vi "ResultsDB Insert Results Data.vi"(6 "Results NameList":string, 7 "Total_OK/NG":string, 8 "error in (no error)":errorcluster, 9 "Results List":string, 10 "StationName":string, 11 "MainBarcode":string) -> (0 "error out":errorcluster, 3 "CMD":string)   [LabVIEW 2021, in "SQLite.lvclass"]
doc: "写入每一步的测试结果到Results表格。\n写入原理：先检测已经保存了几个结果数据，然后依次附加到结果数据列上。\n# 2020-6-8 14:05:45"
uses:
  SQLite.lvclass
  Y:/UTP_2023/Source_Public/DataBase/Top DB/Top DB.lvclass
  <vilib>/Utility/error.llb/Trim Whitespace.vi
  SQLite.lvclass/SQLite.ctl
  <userlib>/LabSQL/LabSQL.lvlib
  vi.lib_New/TopPath/TopPath.lvlib
  <userlib>/sushu/sushu.lvlib
panel:
  out "Update CMD 3":string
  out "Update CMD 2":string
  out "Update CMD":string
  out "EmptyResultColumnIndex":i32
  out "FirstRow":string[](array[string])
  out "source":string
  out "match substring":string
  out "number (0 to 1)":dbl
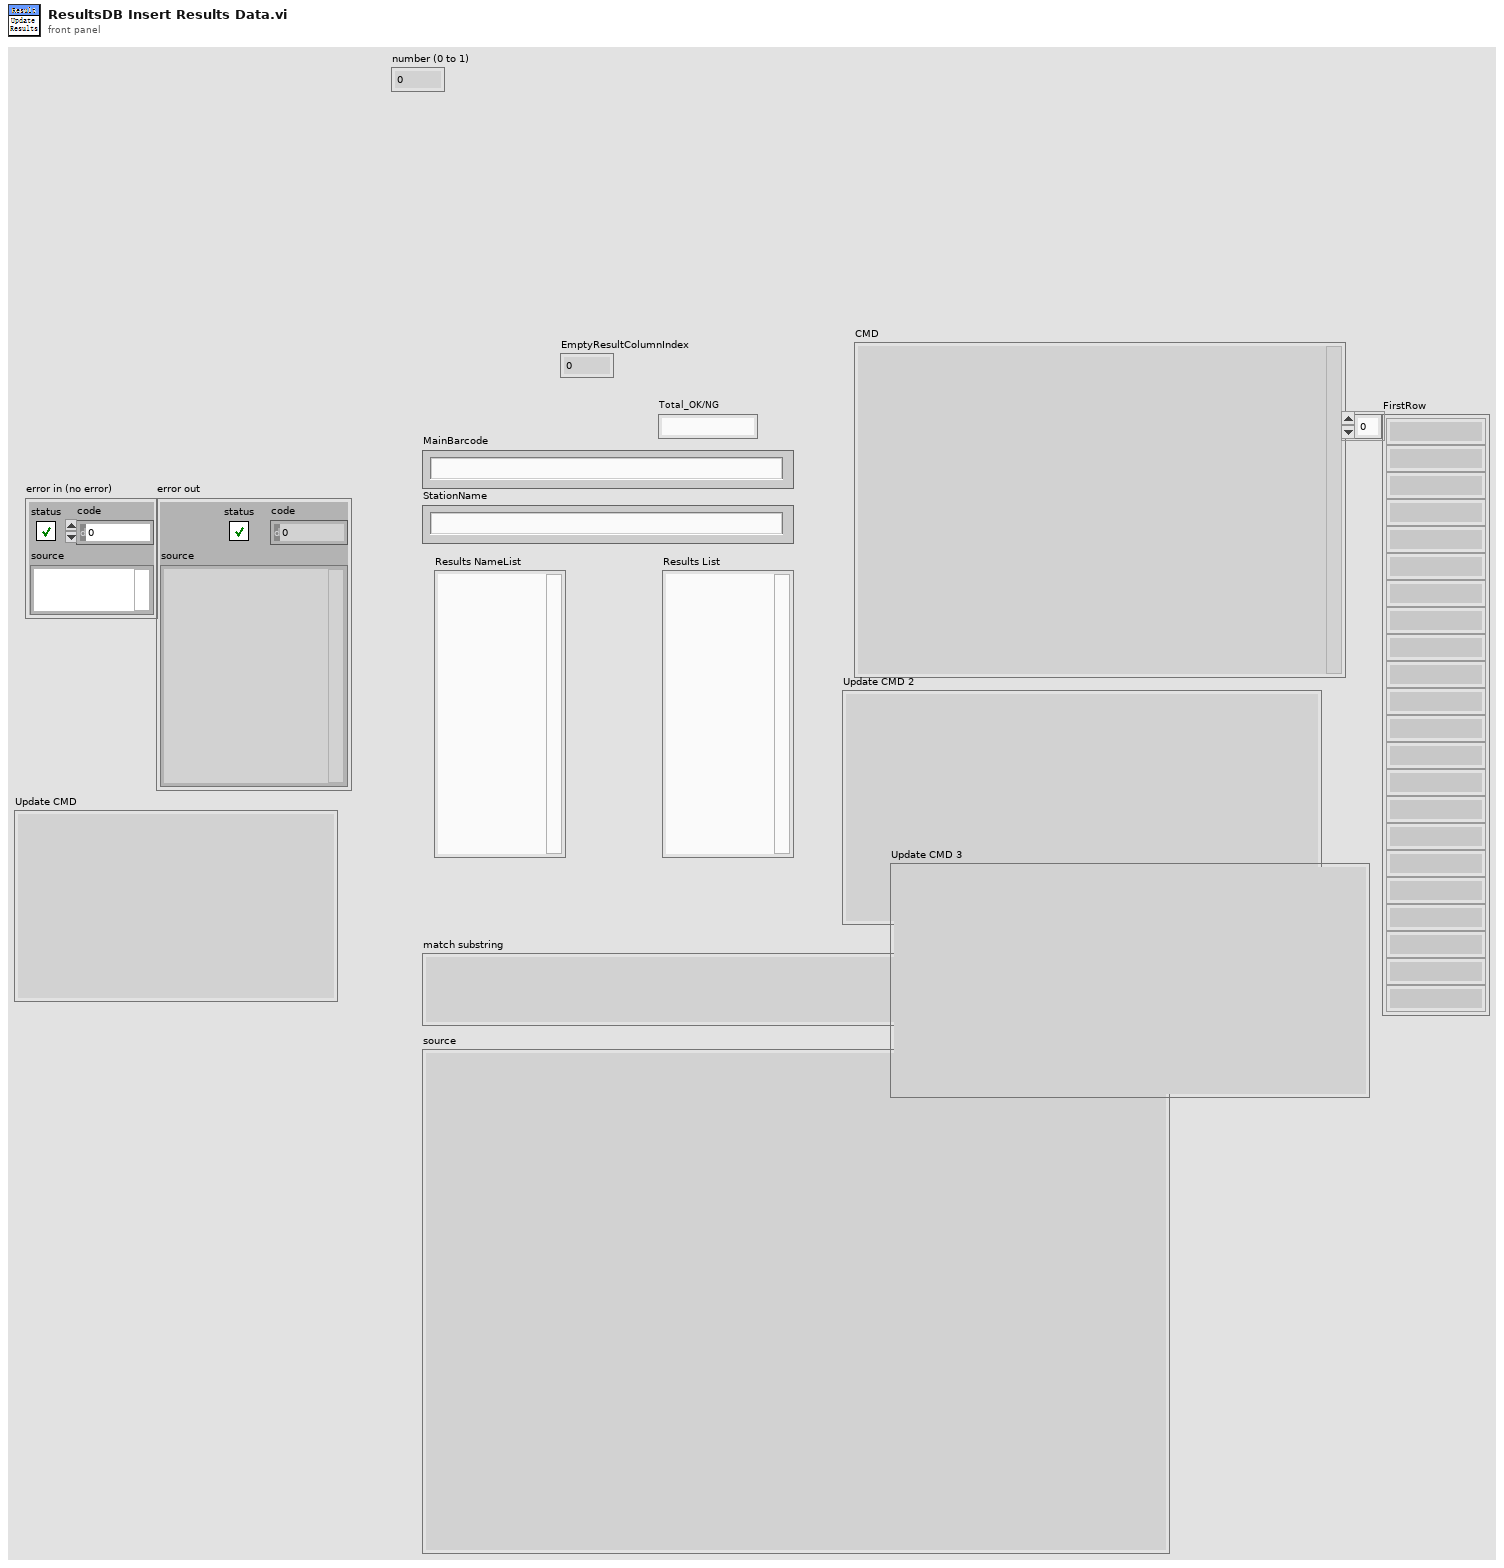
[diagram p1: front panel]
types:
  T1 = cluster{"Core":cluster{"Current VI Reference":refnum<vi>, "Close Panel on Exit?":bool}, "VI Name":string, "Row Numbers":string, "Update?":bool, "CMD":string, "ResultStartindex":i32, "EmptyResultColumnIndex":i32}
  T2 = enum16{"Other", "SQL2008", "SQLite", "Access", "MySQL"}
  T3 = typedef "TopPath.lvlib/Top Path.ctl" = cluster{"LV Source":path, "FilePath":path, "Data":path}
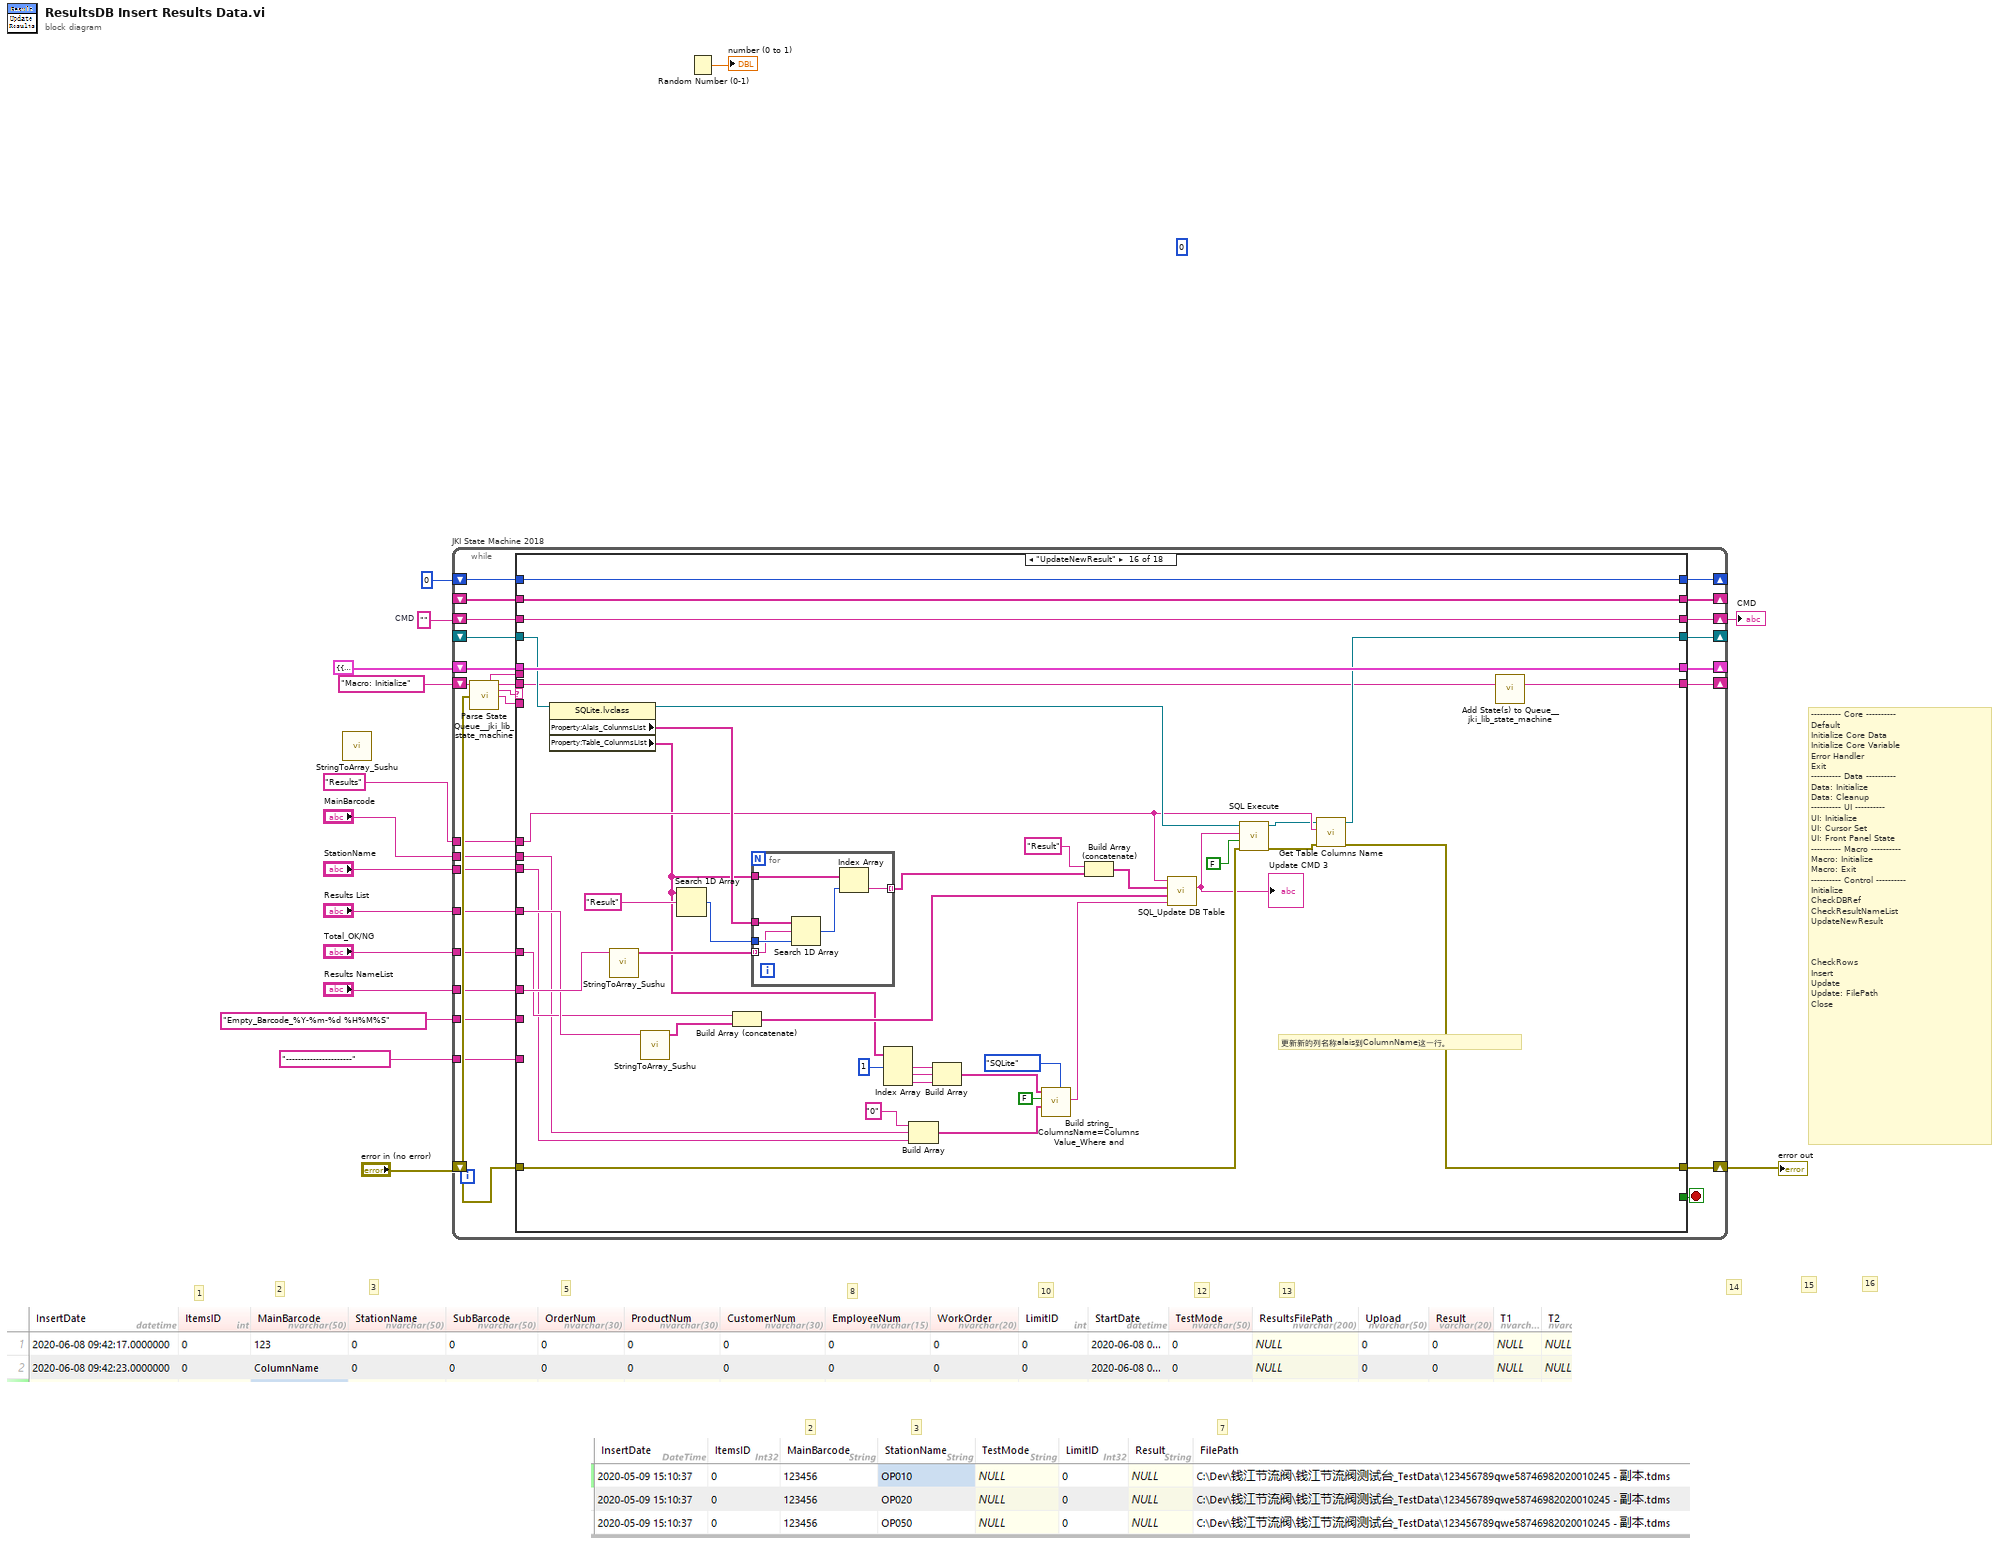
[diagram p0: block diagram]
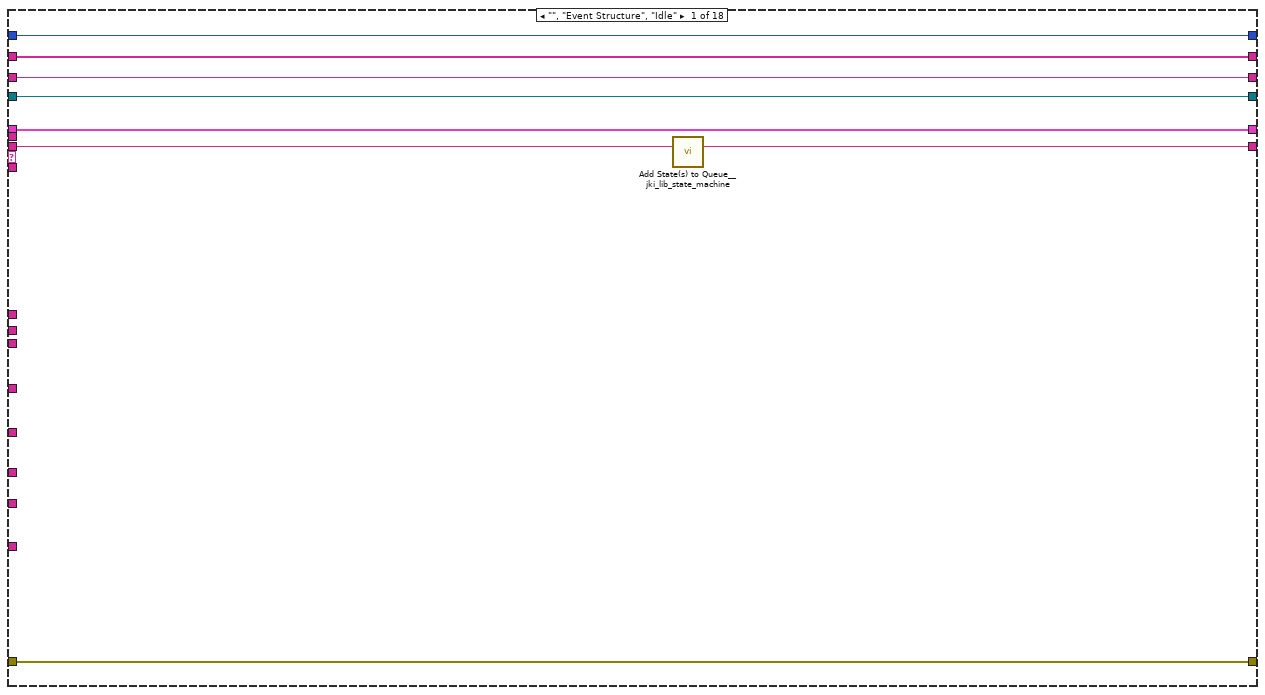
[diagram p2: hidden frame]
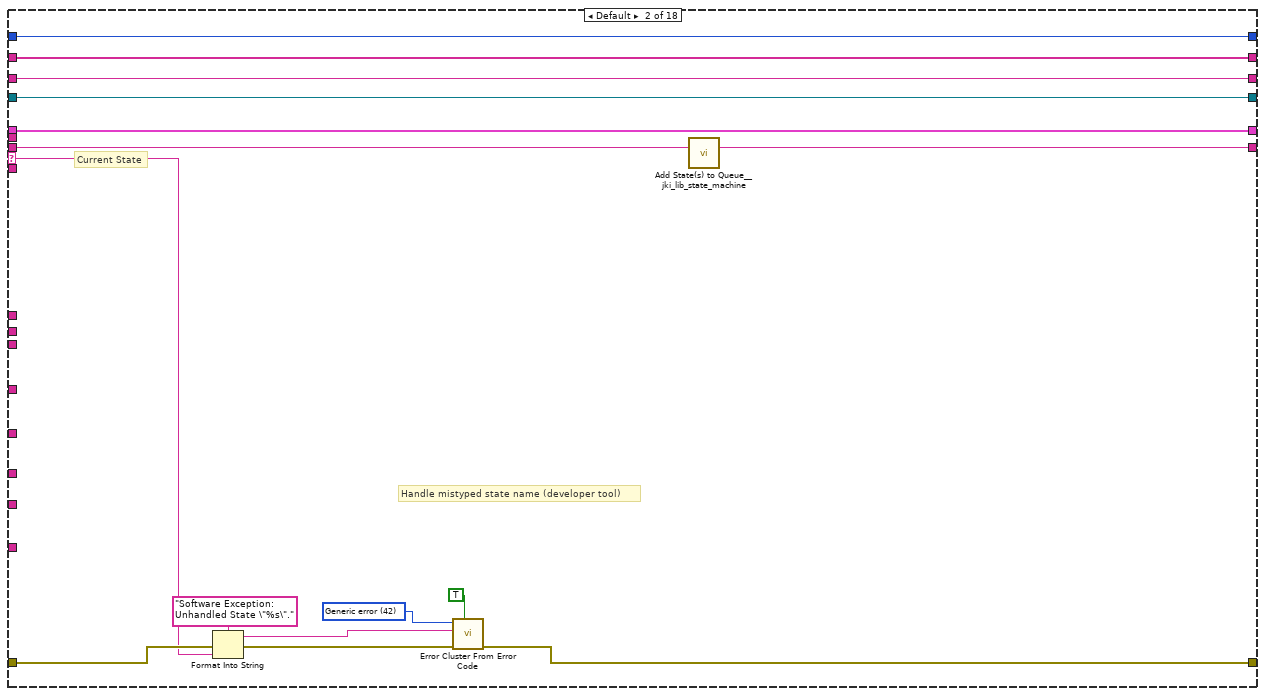
[diagram p3: hidden frame]
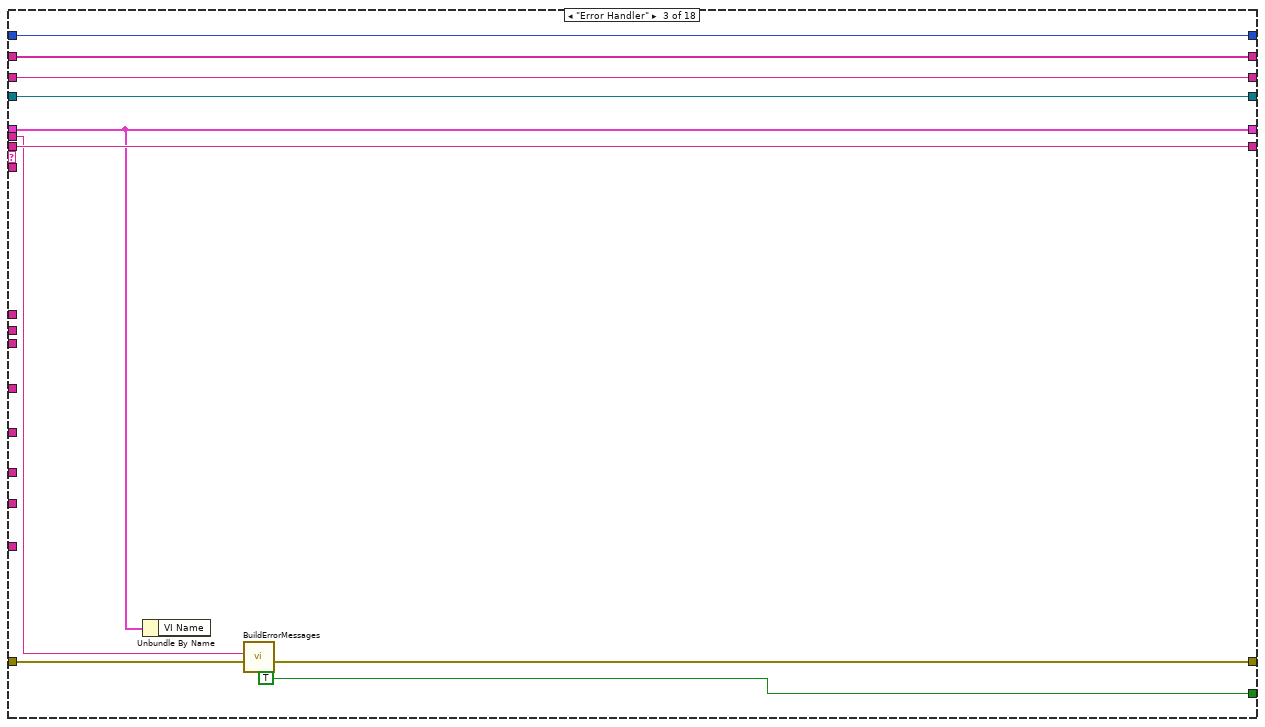
[diagram p4: hidden frame]
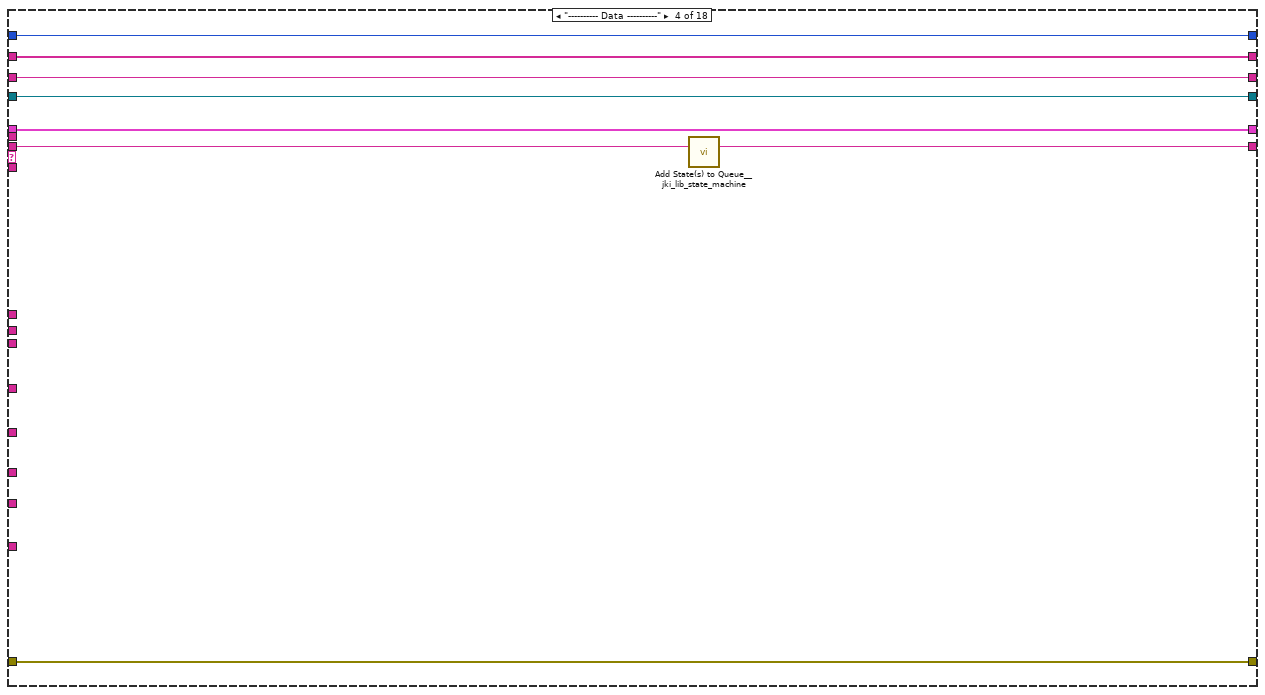
[diagram p5: hidden frame]
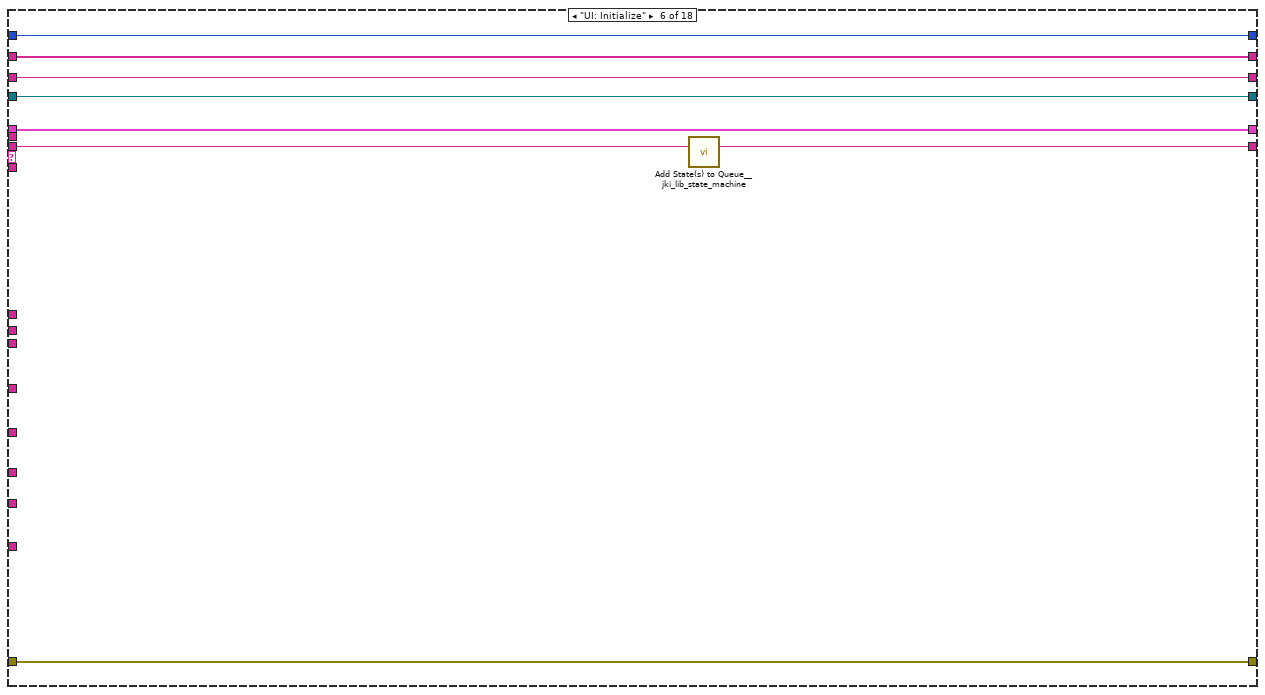
[diagram p7: hidden frame]
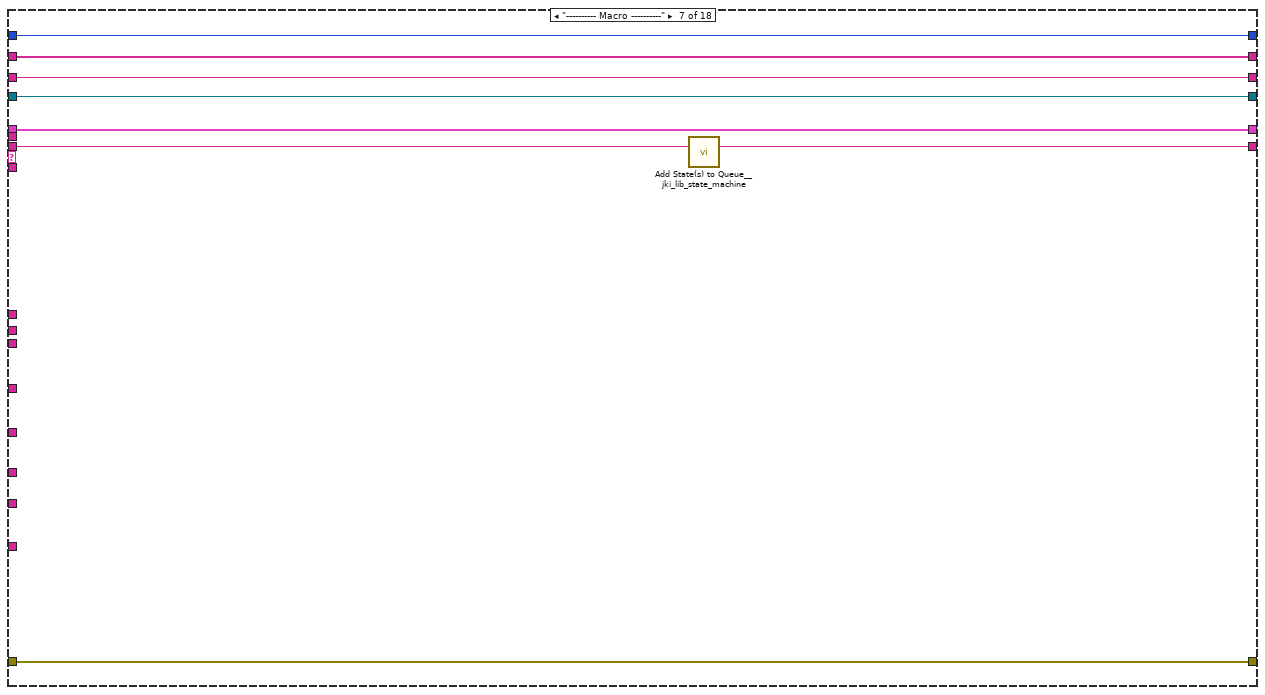
[diagram p8: hidden frame]
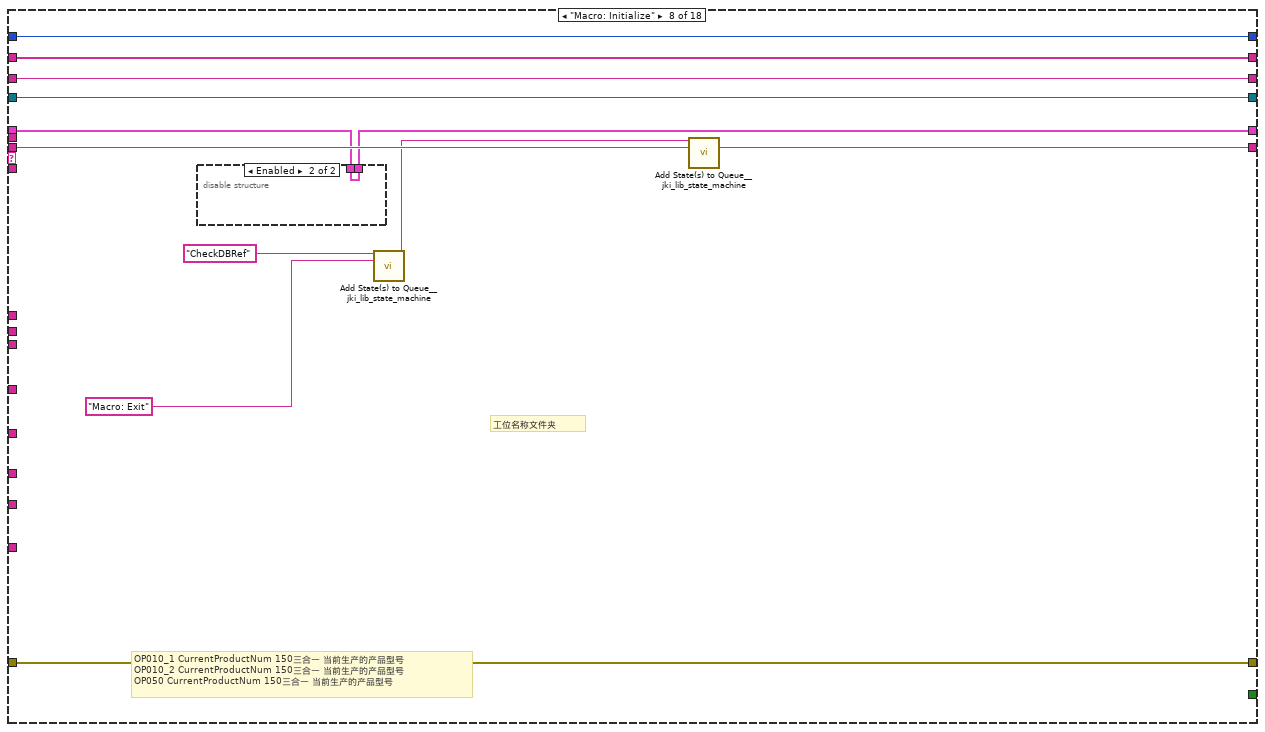
[diagram p9: hidden frame]
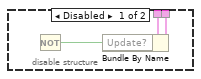
[diagram p10: hidden frame]
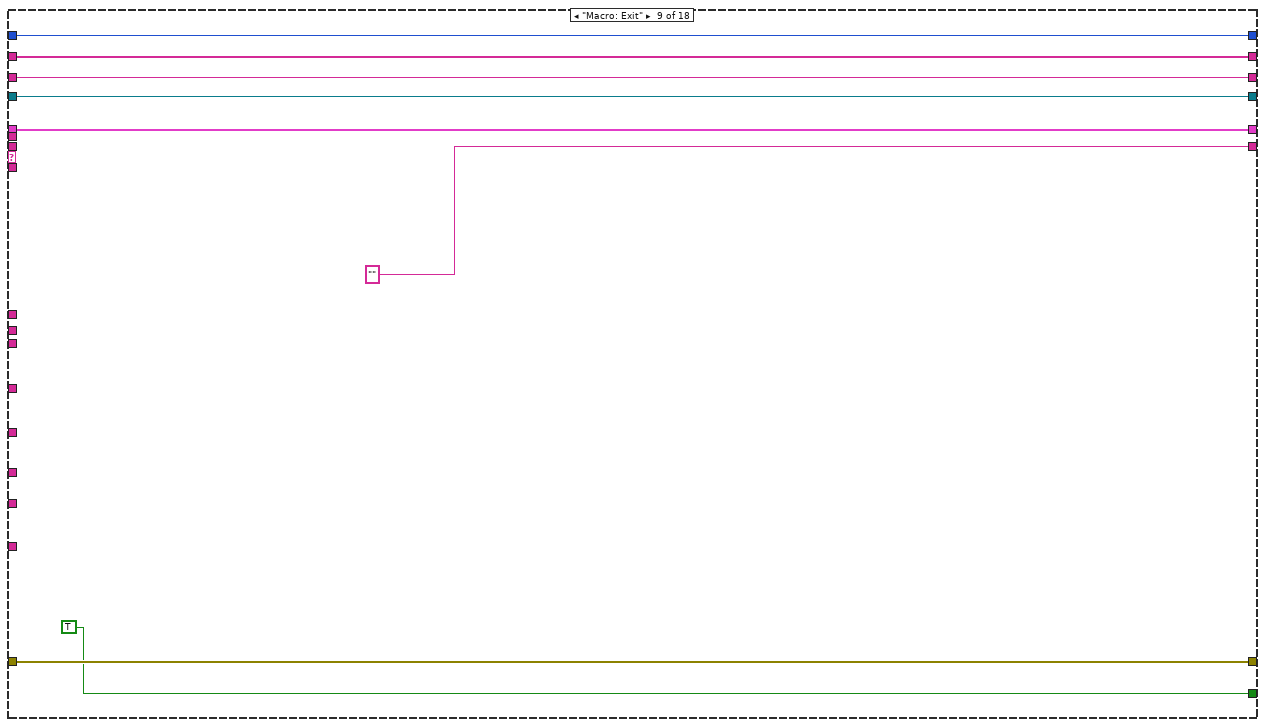
[diagram p11: hidden frame]
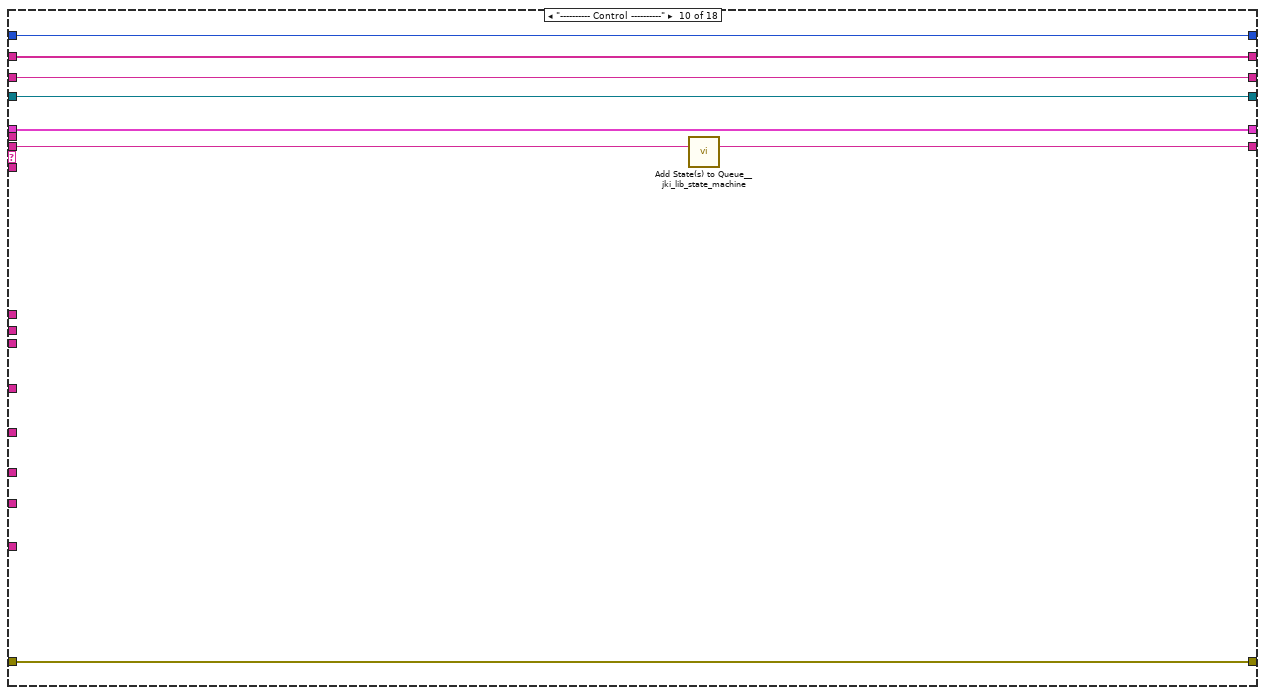
[diagram p12: hidden frame]
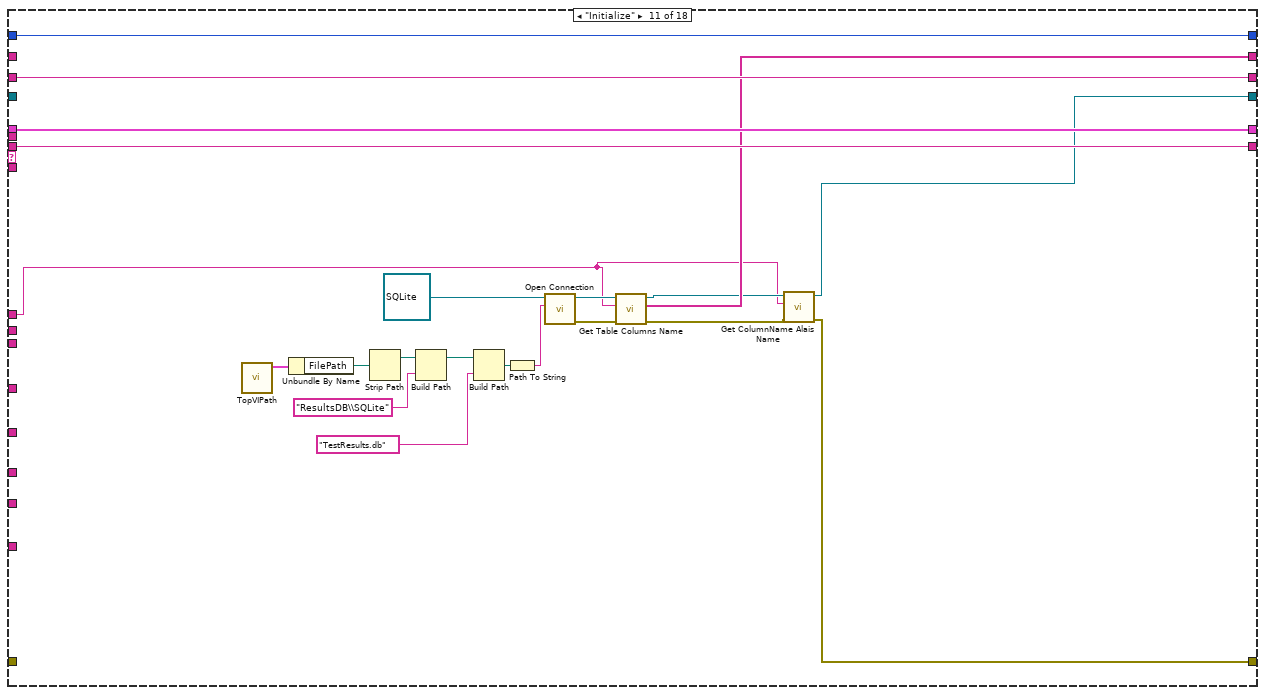
[diagram p13: hidden frame]
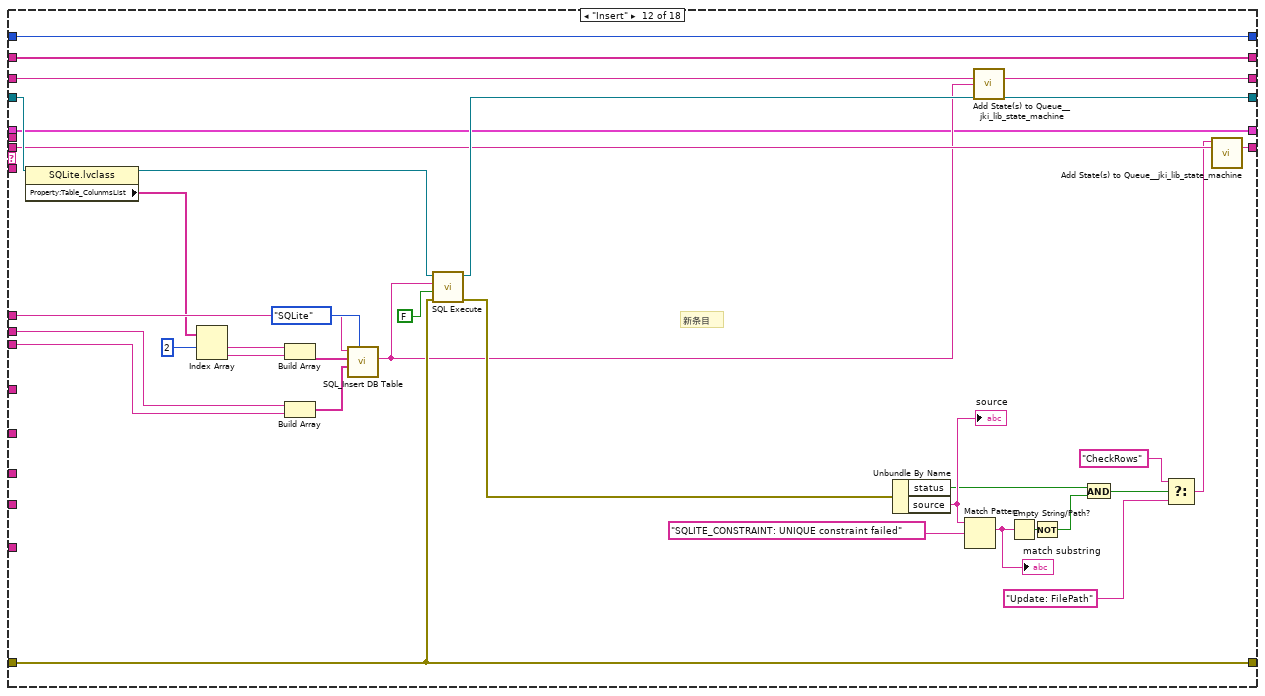
[diagram p14: hidden frame]
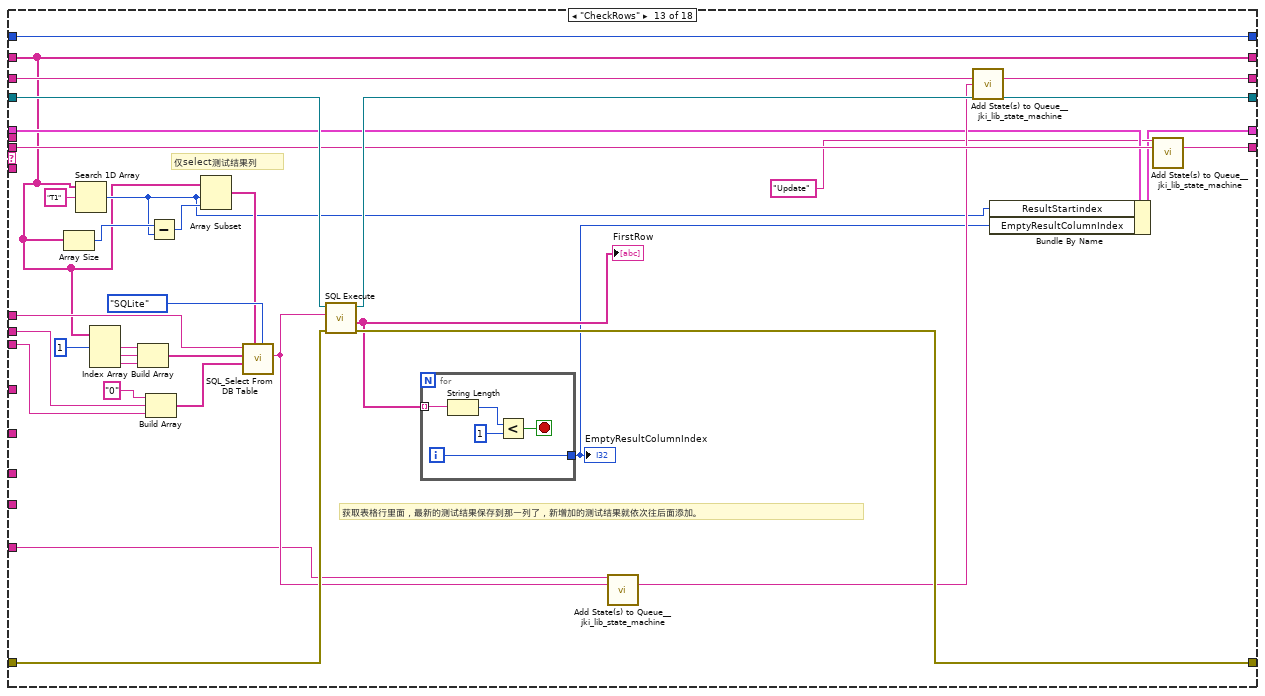
[diagram p15: hidden frame]
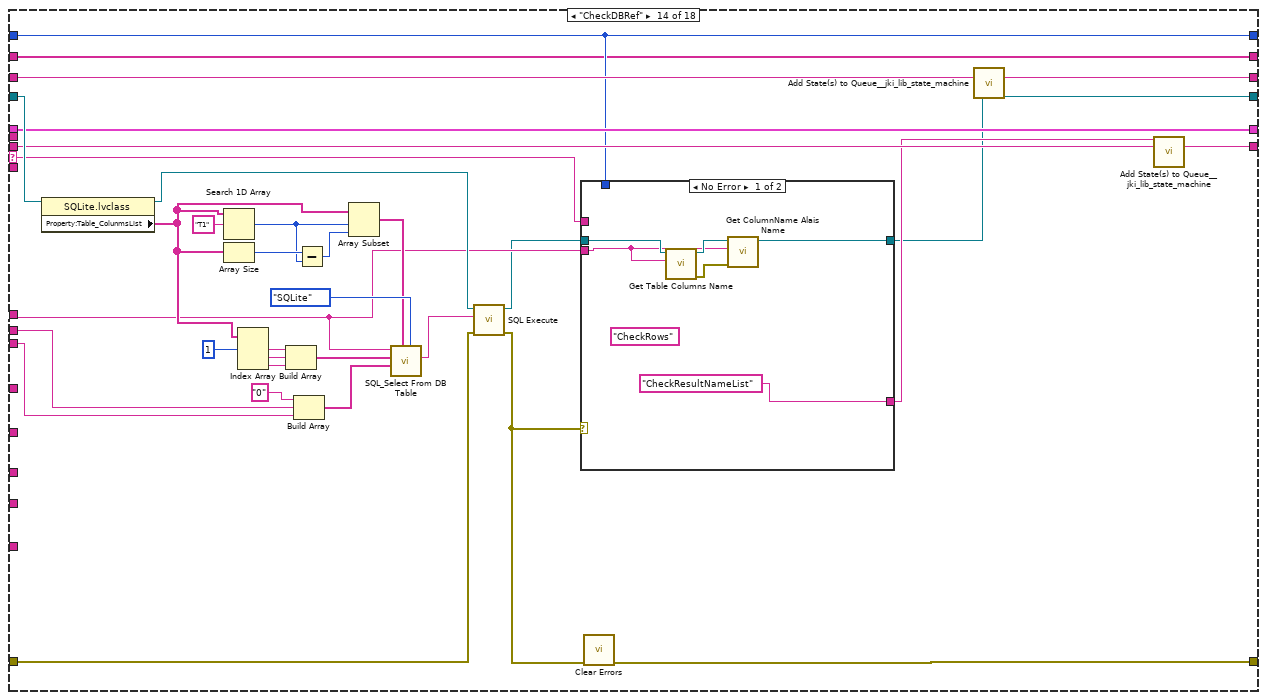
[diagram p16: hidden frame]
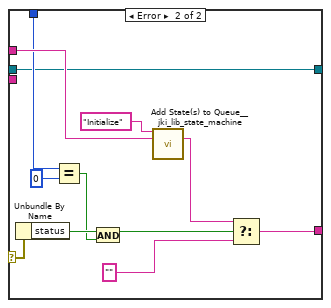
[diagram p17: hidden frame]
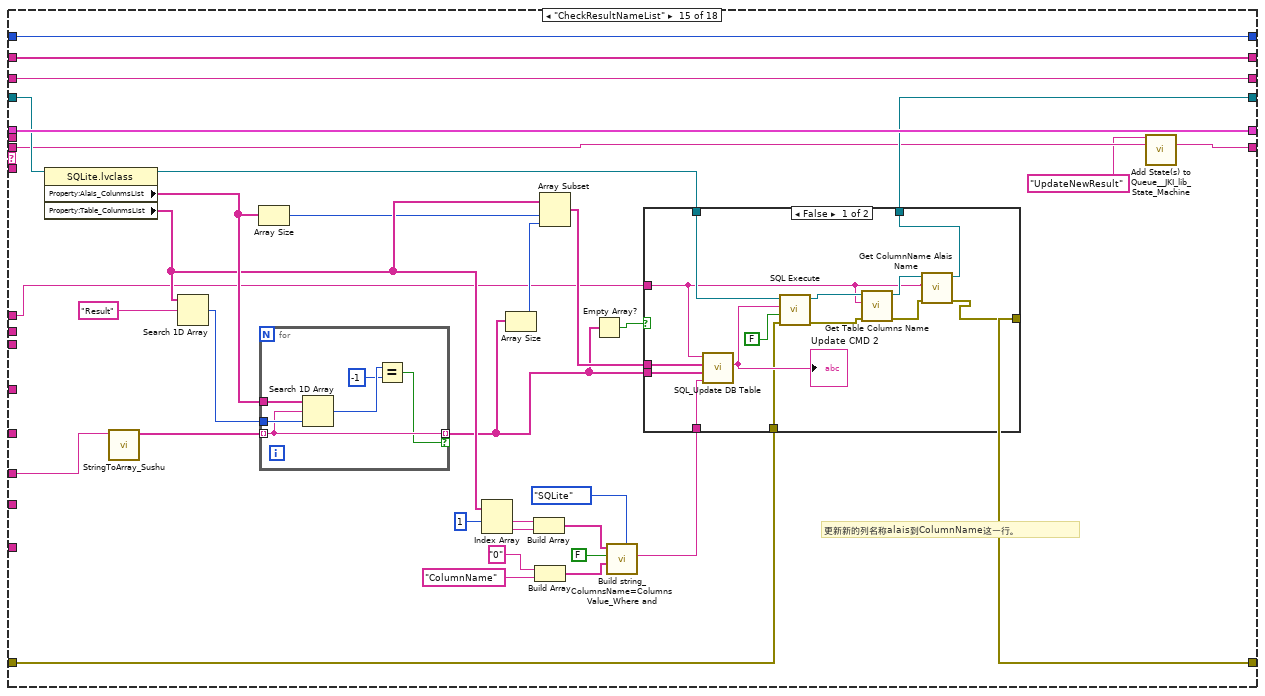
[diagram p18: hidden frame]
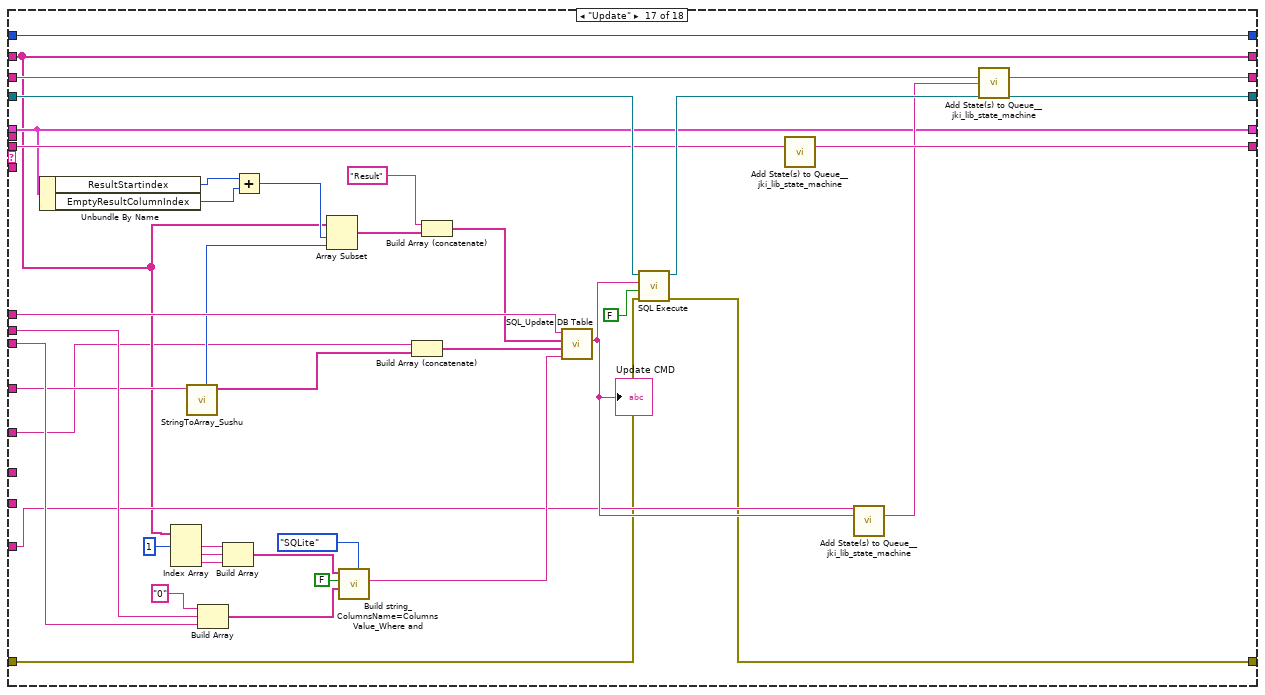
[diagram p20: hidden frame]
diagram:
  w9 = ""  # CMD
  (unwired) 0 ("index (row)")
  # "16"
  # "15"
  # "14"
  # "13"
  # "12"
  # "10"
  # "8"
  # "5"
  # "3"
  # "2"
  # "1"
  # "---------- Core ----------\nDefault\nInitialize Core Data\nInitialize Core Variable\nError Handler\nExit\n---------- Data ----------\nData: Initialize\nData: Cleanup\n---------- UI ----------\nUI: Initialize\nUI: Cursor Set\nUI: Front Panel State\n---------- Macro ----------\nMacro: Initialize\nMacro: Exit\n---------- Control ----------\nInitialize\nCheckDBRef\nCheckResultNameList\nUpdateNewResult\n\n\n\nCheckRows\nInsert\nUpdate\nUpdate: FilePath\nClose"
  # "7"
  # "3"
  # "2"
  n1 = call <userlib>:"StringToArray_Sushu.vi"() -> ()  [unwired: 8 in, 4 out]
  n2 = while "JKI State Machine 2018" {
    shift-right: [w37] -> _
    shift-left: T1 {"Core"={"Current VI Reference"=refnum, "Close Panel on Exit?"=FALSE}, "VI Name"="", "Row Numbers"="", "Update?"=FALSE, "CMD"="", "ResultStartindex"=0, "EmptyResultColumnIndex"=0} ("Data") -> [w36]
    shift-right: [w40] -> w3
    shift-left: "error in (no error)" -> [w35]
    shift-right: [w39] -> _
    shift-left: "Macro: Initialize" -> [w41]
    shift-right: [w33] -> _
    shift-left: _ -> [w34]
    tunnel: "StationName" -> [w31]
    tunnel: "MainBarcode" -> [w30]
    tunnel: "Results" ("TableName") -> [w29]
    tunnel: "Empty_Barcode_%Y-%m-%d %H%M%S" ("time format string (%c)") -> [w28]
    shift-right: [w27] -> w7
    shift-left: w9 -> [w26]
    tunnel: "----------------------" ("State(s) in (\"\")") -> [w25]
    tunnel: "Results List" -> [w24]
    shift-right: [w22] -> _
    shift-left: _ -> [w23]
    shift-right: [w21] -> _
    shift-left: 0 ("y") -> [w20]
    tunnel: "Total_OK/NG" -> [w19]
    tunnel: "Results NameList" -> [w17]
    stop <- w38 stop-if-true
    n3 = call <vilib>:"Parse State Queue__jki_lib_state_machine.vi"("State Queue"=w41, "Error In (no error)"=w35) -> ("Previous State"=w18:string, "Remaining States"=w43:string, "Current State"=w32:string, "Arguments"=w42:string)  [unwired: 10 in]
    n4 = case shown="\"UpdateNewResult\"" w32 {
      selector: w32 -> [_ w56 _ _ _ _ _ _ _ _ _ _ _ w244 _ _ _ _]
      tunnel: w43 -> [w51 w60 w75 w84 w88 w99 w107 w119 _ w139 w160 w172 w216 w257 w287 w366 w420 w436]
      tunnel: w42 -> [_ _ _ _ _ _ _ _ _ _ _ _ _ _ _ _ _ _]
      tunnel: w36 -> [w48 w58 w73 w81 w89 w97 w104 w115 w130 w136 w159 w165 w202 w246 w319 w382 w403 w435]
      tunnel: [w49 w62 w70 w82 w91 w96 w105 w116 w131 w137 w140 w182 w214 w240 w292 w369 w395 w430] -> w40
      tunnel: w35 -> [w49 w61 w71 w82 w91 w96 w105 w116 w131 w137 _ w182 w215 w256 w310 w373 w396 w431]
      tunnel: [w50 w59 w75 w83 w88 w98 w106 w118 "" w138 w160 w173 w217 w258 w288 w367 w421 w436] -> w39
      tunnel: [_ _ TRUE _ _ _ _ _ TRUE _ _ _ _ _ _ _ _ _] -> w38
      tunnel: [w48 w58 w73 w81 w89 w97 w104 w111 w130 w136 w159 w165 w199 w246 w319 w382 w403 w435] -> w37
      tunnel: w34 -> [w47 w55 w74 w80 w90 w95 w103 w117 w129 w135 _ w185 w219 w259 w318 w381 w424 w429]
      tunnel: [w47 w55 w74 w80 w90 w95 w103 w117 w129 w135 w143 w184 w218 w234 w293 w370 w423 w428] -> w33
      tunnel: w18 -> [_ _ w72 _ _ _ _ _ _ _ _ _ _ _ _ _ _ _]
      tunnel: w31 -> [_ _ _ _ _ _ _ _ _ _ _ w186 w220 w260 _ w342 w425 _]
      tunnel: w30 -> [_ _ _ _ _ _ _ _ _ _ _ w187 w221 w261 _ w343 w426 _]
      tunnel: w29 -> [_ _ _ _ _ _ _ _ _ _ w142 w188 w222 w236 w291 w368 w427 _]
      tunnel: w28 -> [_ _ _ _ _ _ _ _ _ _ _ _ _ _ _ _ _ _]
      tunnel: w26 -> [w46 w54 w69 w79 w87 w94 w102 w112 w126 w134 w158 w168 w212 w254 w317 w380 w408 w434]
      tunnel: [w46 w54 w69 w79 w87 w94 w102 w112 w126 w134 w158 w167 w213 w255 w317 w380 w409 w434] -> w27
      tunnel: w25 -> [_ _ _ _ _ _ _ _ _ _ _ _ w209 _ _ _ w405 _]
      tunnel: w24 -> [_ _ _ _ _ _ _ _ _ _ _ _ _ _ _ w361 w404 _]
      tunnel: w23 -> [w45 w53 w68 w78 w86 w93 w101 w109 w125 w133 _ w162 w196 w238 w316 w379 w394 w433]
      tunnel: [w45 w53 w68 w78 w86 w93 w101 w109 w125 w133 w145 w162 w196 w238 w316 w379 w394 w433] -> w22
      tunnel: w20 -> [w44 w52 w67 w77 w85 w92 w100 w108 w124 w132 w146 w164 w195 w243 w315 w378 w393 w432]
      tunnel: [w44 w52 w67 w77 w85 w92 w100 w108 w124 w132 w146 w164 w195 w243 w315 w378 w393 w432] -> w21
      tunnel: w19 -> [_ _ _ _ _ _ _ _ _ _ _ _ _ _ _ w359 w391 _]
      tunnel: w17 -> [_ _ _ _ _ _ _ _ _ _ _ _ _ _ w294 w371 _ _]
      frame "", "Event Structure", "Idle" {
        n5 = call <vilib>:"Add State(s) to Queue__jki_lib_state_machine.vi"("State(s) in (\"\")"=w51) -> ("States Out"=w50:string)  [unwired: 14 in]
      }
      frame Default {
        w65 = 42 items=["No error", "Argument error", "Memory is full", "Out of zone", "End of file", "File already open", "Generic file I/O error", "File not found", "File permission error", "Disk is full", "Duplicate path", "Too many files open", "System feature not enabled", "Resource file not found", "Cannot add resource", "Resource not found", "Image not found", "Image memory error", "Pen does not exist", "Config type invalid", "Config token not found", "Config parse error", "Config memory error", "Bad external code format", "Bad external code offset", "External code not present", "Null window", "Destroy window error", "Null menu", "Print aborted", "Bad print record", "Print driver error", "Windows error during printing", "Memory error during printing", "Print dialog error", "Generic print error", "Invalid device refnum", "Device not found", "Device parameter error", "Device unit error", "Cannot open device", "Device call aborted", "Generic error", "Cancelled by user", "Object ID too low", "Object ID too high", "Object not in heap", "Unknown heap", "Unknown object (invalid DefProc)", "Unknown object (DefProc not in table)", "Message out of range", "Invalid (null) method", "Unknown message", "Manager call not supported", "Bad address", "Network operation in progress", "Network operation timed out", "Connection is busy", "Network attribute not supported", "Network error", "Address in use", "System out of memory", "Connection aborted", "Connection refused", "Not connected", "Already connected", "Connection closed", "Initialization error (interapplication manager)", "Bad occurrence", "Wait on unbound occurrence handler", "Occurrence queue overflow", "Datalog type conflict", "Unused", "Unrecognized type (interapplication manager)", "Memory corrupt", "Failed to make temporary DLL", "Old CIN version", "Drag socket not found", "Failed to load drop-object", "Failed to register OLE object", "Failed to release OLE object", "Format specifier type mismatch", "Unknown format specifier", "Too few format specifiers", "Too many format specifiers", "Scan failed", "Newer CIN version", "Error converting to variant", "Runtime menu error", "Password tampered", "Variant attribute not found", "Incompatible variant data type", "Event data is not available", "Event Store is not present", "Occurrence is not found", "Event Queue is not created", "Event info is not available", "Refnum passed is NULL", "Error retrieving Class GUID", "Error retrieving CoClass GUID", "Error retrieving TypeLib GUID.", "Bad built application magic bytes.", "Specific driver is different from the specific driver associated with the Logical Name.", "There is no session opened to the class driver.", "Max Error", "MAX - Error with config objects", "MAX - Error loading configuration", "MAX - Group not supported"]
        # "Current State"
        # "Handle mistyped state name (developer tool)"
        n6 = Format Into String(format string="Software Exception: Unhandled State \"%s\"." ("message"), error in=w61, w56) -> (resulting string=w64:string, error out=w63:errorcluster)  [unwired: 1 in]
        n7 = call <vilib>:"Error Cluster From Error Code.vi"("show call chain? (False)"=TRUE, "error in (no error)"=w63, "error message (\"\")"=w64, "error code (0)"=w65) -> ("error out"=w62:errorcluster)  [unwired: 5 in]
        n8 = call <vilib>:"Add State(s) to Queue__jki_lib_state_machine.vi"("State(s) in (\"\")"=w60) -> ("States Out"=w59:string)  [unwired: 14 in]
      }
      frame "Error Handler" {
        n9 = Unbundle By Name(w73) -> ()  [unwired: 1 out]
        n10 = call <userlib>:"BuildErrorMessages.vi"("error in"=w71, "ErrorCase"=w72) -> ("error out (no error)"=w70:errorcluster)  [unwired: 7 in, 2 out]
      }
      frame "---------- Data ----------" {
        n11 = call <vilib>:"Add State(s) to Queue__jki_lib_state_machine.vi"("State(s) in (\"\")"=w84) -> ("States Out"=w83:string)  [unwired: 14 in]
      }
      frame "Data: Initialize" {
      }
      frame "UI: Initialize" {
        n12 = call <vilib>:"Add State(s) to Queue__jki_lib_state_machine.vi"("State(s) in (\"\")"=w99) -> ("States Out"=w98:string)  [unwired: 14 in]
      }
      frame "---------- Macro ----------" {
        n13 = call <vilib>:"Add State(s) to Queue__jki_lib_state_machine.vi"("State(s) in (\"\")"=w107) -> ("States Out"=w106:string)  [unwired: 14 in]
      }
      frame "Macro: Initialize" {
        # "OP010_1\tCurrentProductNum\t150三合一\t当前生产的产品型号\nOP010_2\tCurrentProductNum\t150三合一\t当前生产的产品型号\nOP050\tCurrentProductNum\t150三合一\t当前生产的产品型号"
        # "工位名称文件夹"
        n14 = disable-structure shown="Enabled" {
          disable-tunnel: w115 -> [w122 w123]
          disable-tunnel: [w121 w123] -> w111
          frame Disabled {
            n15 = Not() -> (.not. x?=w120:bool)  [unwired: 1 in]
            n16 = Bundle By Name(cluster=w122, "Update?"=w120) -> (w121:T1)
          }
          frame Enabled {
          }
        }
        n17 = call <vilib>:"Add State(s) to Queue__jki_lib_state_machine.vi"("State(s) in Front (\"\")"="CheckDBRef" ("State(s) in Front (\"\")"), "State(s) in (\"\")"="Macro: Exit") -> ("States Out"=w114:string)  [unwired: 13 in]
        n18 = call <vilib>:"Add State(s) to Queue__jki_lib_state_machine.vi"("State(s) in Front (\"\")"=w114, "State(s) in (\"\")"=w119) -> ("States Out"=w118:string)  [unwired: 13 in]
      }
      frame "Macro: Exit" {
      }
      frame "---------- Control ----------" {
        n19 = call <vilib>:"Add State(s) to Queue__jki_lib_state_machine.vi"("State(s) in (\"\")"=w139) -> ("States Out"=w138:string)  [unwired: 14 in]
      }
      frame "Initialize" {
        n20 = call "TopVIPath.vi"() -> ("TopPath"=w147:T3)  [unwired: 10 in, 1 out]
        n21 = Unbundle By Name(w147) -> ("FilePath"=w157:path)
        n22 = Strip Path(path=w157) -> (stripped path=w156:path)  [unwired: 1 out]
        n23 = Build Path(base path=w156, name or relative path="ResultsDB\\SQLite") -> (appended path=w154:path)
        n24 = Build Path(base path=w154, name or relative path="TestResults.db") -> (appended path=w152:path)
        n25 = Path To String(path=w152) -> (string=w151:string)
        n26 = call-dynamic "Open Connection.vi"("ConnectionString"=w151, "HostDB in"=refnum<class "SQLite.lvclass"> refnum ("SQLite.lvclass")) -> ("error out"=w149:errorcluster, "HostDB out"=w150:refnum<class "SQLite.lvclass">)  [unwired: 8 in]
        n27 = call-dynamic "Get Table Columns Name.vi"("error in (no error)"=w149, "TableName"=w142, "HostDB in"=w150) -> ("error out"=w141:errorcluster, "Table_ColunmsList"=w145:string[], "HostDB out"=w144:refnum<class "SQLite.lvclass">)  [unwired: 4 in, 2 out]
        n28 = call "Get ColumnName Alais Name.vi"("error in (no error)"=w141, "TableName"=w142, "SQLite in"=w144) -> ("error out"=w140:errorcluster, "SQLite out"=w143:refnum<class "SQLite.lvclass">)  [unwired: 6 in, 1 out]
      }
      frame "Insert" {
        # "新条目"
        n29 = property class="SQLite.lvclass"(reference=w185) -> (reference out=w163:refnum<class "SQLite.lvclass">, "Property:Table_ColunmsList"=w161:string[])  [unwired: 1 in, 1 out]
        n30 = Index Array(array=w161, index #1=2 ("index")) -> (element #1=w193:string, element #2=w194:string)  [unwired: 1 in]
        n31 = Build Array(w193, w194) -> (w191:string[])
        n32 = Build Array(w187, w186) -> (w190:string[])
        n33 = call <userlib>:"SQL_Insert DB Table.vi"("DB Type"=T2."SQLite", "ColumnsValue"=w190, "ColumnsName"=w191, "Table Name"=w188) -> ("Insert DB String"=w166:string)  [unwired: 7 in]
        n34 = call-dynamic "SQL Execute.vi"("error in (no error)"=w182, "Return Data (T)"=FALSE, "Command Text"=w166, "HostDB in"=w163) -> ("error out"=w169:errorcluster, "HostDB out"=w184:refnum<class "SQLite.lvclass">)  [unwired: 3 in, 3 out]
        n35 = Unbundle By Name(w169) -> ("status"=w178:bool, "source"=w181:string)
        "source" <- w181
        n36 = Match Pattern(string=w181, regular expression="SQLITE_CONSTRAINT: UNIQUE constraint failed") -> (match substring=w179:string)  [unwired: 1 in, 3 out]
        "match substring" <- w179
        n37 = call <vilib>:"Add State(s) to Queue__jki_lib_state_machine.vi"("State(s) in (\"\")"=w168, "State(s) at Back (\"\")"=w166) -> ("States Out"=w167:string)  [unwired: 13 in]
        n38 = Empty String/Path?(string/path=w179) -> (empty?=w177:bool)
        n39 = Not(x=w177) -> (.not. x?=w170:bool)
        n40 = And(x=w178, y=w170) -> (x .and. y?=w176:bool)
        n41 = Select(t="CheckRows", s=w176, f="Update: FilePath") -> (s? t:f=w171:string)
        n42 = call <vilib>:"Add State(s) to Queue__jki_lib_state_machine.vi"("State(s) in Front (\"\")"=w171, "State(s) in (\"\")"=w172) -> ("States Out"=w173:string)  [unwired: 13 in]
      }
      frame "CheckRows" {
        # "获取表格行里面，最新的测试结果保存到那一列了，新增加的测试结果就依次往后面添加。"
        # "仅select测试结果列"
        n43 = Array Size(array=w196) -> (size(s)=w205:i32)
        n44 = Search 1D Array(1D array=w196, element="T1") -> (index of element=w198:i32)  [unwired: 1 in]
        n45 = Index Array(array=w196, index #1=1 ("index")) -> (element #1=w227:string, element #2=w228:string, element #3=w208:string)  [unwired: 2 in]
        n46 = Build Array(w227, w228, w208) -> (w225:string[])
        n47 = Build Array("0" ("element"), w221, w220) -> (w224:string[])
        n48 = Subtract(x=w205, y=w198) -> (x-y=w204:i32)
        n49 = Array Subset(array=w196, index=w198, length=w204) -> (w203:string[])
        n50 = call <userlib>:"SQL_Select From DB Table.vi"("DB Type"=T2."SQLite", "SelectedColumnsNameList"=w203, "ColumnsValue"=w224, "ColumnsNameList"=w225, "TableName"=w222) -> ("Select SQL CMD"=w210:string)  [unwired: 6 in]
        n51 = call-dynamic "SQL Execute.vi"("error in (no error)"=w215, "Command Text"=w210, "HostDB in"=w219) -> ("error out"=w214:errorcluster, "FirstRow"=w201:string[], "HostDB out"=w218:refnum<class "SQLite.lvclass">)  [unwired: 4 in, 2 out]
        "FirstRow" <- w201
        n52 = for {
          tunnel: w201 -> [w233] mode=indexing
          tunnel: [w229] -> w197
          i -> [w229]
          stop <- w230 stop-if-true
          n53 = String Length(string=w233) -> (length=w232:i32)
          n54 = Less?(x=w232, y=1) -> (x < y?=w230:bool)
        }
        "EmptyResultColumnIndex" <- w197
        n55 = call <vilib>:"Add State(s) to Queue__jki_lib_state_machine.vi"("State(s) in Front (\"\")"=w209, "State(s) in (\"\")"=w210) -> ("States Out"=w211:string)  [unwired: 13 in]
        n56 = call <vilib>:"Add State(s) to Queue__jki_lib_state_machine.vi"("State(s) in (\"\")"=w212, "State(s) at Back (\"\")"=w211) -> ("States Out"=w213:string)  [unwired: 13 in]
        n57 = Bundle By Name(cluster=w202, "ResultStartindex"=w198, "EmptyResultColumnIndex"=w197) -> (w199:T1)
        n58 = call <vilib>:"Add State(s) to Queue__jki_lib_state_machine.vi"("State(s) in Front (\"\")"="Update" ("State(s) in Front (\"\")"), "State(s) in (\"\")"=w216) -> ("States Out"=w217:string)  [unwired: 13 in]
      }
      frame "CheckDBRef" {
        n59 = property class="SQLite.lvclass"(reference=w259) -> (reference out=w239:refnum<class "SQLite.lvclass">, "Property:Table_ColunmsList"=w237:string[])  [unwired: 1 in, 1 out]
        n60 = Search 1D Array(1D array=w237, element="T1") -> (index of element=w247:i32)  [unwired: 1 in]
        n61 = Array Size(array=w237) -> (size(s)=w249:i32)
        n62 = Index Array(array=w237, index #1=1 ("index")) -> (element #1=w266:string, element #2=w267:string, element #3=w252:string)  [unwired: 2 in]
        n63 = Build Array(w266, w267, w252) -> (w264:string[])
        n64 = Build Array("0" ("element"), w261, w260) -> (w263:string[])
        n65 = Subtract(x=w249, y=w247) -> (x-y=w248:i32)
        n66 = Array Subset(array=w237, index=w247, length=w248) -> (w241:string[])
        n67 = call <userlib>:"SQL_Select From DB Table.vi"("DB Type"=T2."SQLite", "SelectedColumnsNameList"=w241, "ColumnsValue"=w263, "ColumnsNameList"=w264, "TableName"=w236) -> ("Select SQL CMD"=w253:string)  [unwired: 6 in]
        n68 = call-dynamic "SQL Execute.vi"("error in (no error)"=w256, "Command Text"=w253, "HostDB in"=w239) -> ("error out"=w245:errorcluster, "HostDB out"=w235:refnum<class "SQLite.lvclass">)  [unwired: 4 in, 3 out]
        n69 = case shown="No Error" w245 {
          selector: w245 -> [_ w281]
          tunnel: w244 -> [_ w282]
          tunnel: ["CheckResultNameList" ("TableName") w280] -> w242
          tunnel: w243 -> [_ w277]
          tunnel: w235 -> [w271 w274]
          tunnel: w236 -> [w269 _]
          tunnel: [w272 w274] -> w234
          frame No Error {
            (unwired) "CheckRows" ("TableName")
            n70 = call-dynamic "Get Table Columns Name.vi"("TableName"=w269, "HostDB in"=w271) -> ("error out"=w268:errorcluster, "HostDB out"=w270:refnum<class "SQLite.lvclass">)  [unwired: 5 in, 3 out]
            n71 = call "Get ColumnName Alais Name.vi"("error in (no error)"=w268, "TableName"=w269, "SQLite in"=w270) -> ("SQLite out"=w272:refnum<class "SQLite.lvclass">)  [unwired: 6 in, 2 out]
          }
          frame Error {
            n72 = Unbundle By Name(w281) -> ("status"=w279:bool)
            n73 = Equal?(x=w277, y=0) -> (x = y?=w275:bool)
            n74 = And(x=w279, y=w275) -> (x .and. y?=w278:bool)
            n75 = call <vilib>:"Add State(s) to Queue__jki_lib_state_machine.vi"("State(s) in Front (\"\")"="Initialize" ("Remaining States"), "State(s) in (\"\")"=w282) -> ("States Out"=w283:string)  [unwired: 13 in]
            n76 = Select(t=w283, s=w278, f="") -> (s? t:f=w280:string)
          }
        }
        n77 = call <vilib>:"Clear Errors.vi"("error in (no error)"=w245) -> ("error out"=w240:errorcluster)  [unwired: 5 in, 1 out]
        n78 = call <vilib>:"Add State(s) to Queue__jki_lib_state_machine.vi"("State(s) in (\"\")"=w254) -> ("States Out"=w255:string)  [unwired: 14 in]
        n79 = call <vilib>:"Add State(s) to Queue__jki_lib_state_machine.vi"("State(s) in Front (\"\")"=w242, "State(s) in (\"\")"=w257) -> ("States Out"=w258:string)  [unwired: 13 in]
      }
      frame "CheckResultNameList" {
        # "更新新的列名称alais到ColumnName这一行。"
        n80 = property class="SQLite.lvclass"(reference=w318) -> (reference out=w311:refnum<class "SQLite.lvclass">, "Property:Alais_ColunmsList"=w299:string[], "Property:Table_ColunmsList"=w298:string[])  [unwired: 1 in, 1 out]
        n81 = call <userlib>:"StringToArray_Sushu.vi"("State Queue"=w294) -> ("Array"=w314:string[])  [unwired: 7 in, 3 out]
        n82 = Search 1D Array(1D array=w298, element="Result") -> (index of element=w312:i32)  [unwired: 1 in]
        n83 = Array Size(array=w299) -> (size(s)=w297:i32)
        n84 = for {
          tunnel: w314 -> [w337] mode=indexing
          tunnel: w299 -> [w341]
          tunnel: w312 -> [w340]
          tunnel: [w337] -> w290 mode=indexing if=w336
          n85 = Search 1D Array(1D array=w341, element=w337, start index (0)=w340) -> (index of element=w339:i32)
          n86 = Equal?(x=w339, y=-1) -> (x = y?=w336:bool)
        }
        n87 = Index Array(array=w298, index #1=1 ("index")) -> (element #1=w308:string, element #2=w307:string)  [unwired: 1 in]
        n88 = Array Size(array=w290) -> (size(s)=w296:i32)
        n89 = Build Array(w308, w307) -> (w306:string[])
        n90 = Build Array("0" ("element"), "ColumnName" ("element")) -> (w304:string[])
        n91 = Array Subset(array=w298, index=w297, length=w296) -> (w295:string[])
        n92 = Empty Array?(array=w290) -> (empty?=w289:bool)
        n93 = call <userlib>:"Build string_ColumnsName=ColumnsValue_Where and.vi"("DB Type"=T2."SQLite", "ColumnsValue"=w304, "Check ASCII?"=FALSE, "ColumnsNameList"=w306) -> ("ColumnName='ColumnValue'"=w301:string)  [unwired: 7 in]
        n94 = case shown="False" w289 {
          tunnel: w311 -> [w331 w335]
          tunnel: w310 -> [w330 w334]
          tunnel: w301 -> [w329 _]
          tunnel: w295 -> [w328 _]
          tunnel: [w323 w335] -> w293
          tunnel: [w320 w334] -> w292
          tunnel: w291 -> [w322 _]
          tunnel: w290 -> [w325 _]
          frame False {
            n95 = call <userlib>:"SQL_Update DB Table.vi"("where name='value'"=w329, "ColumnsValue"=w325, "ColumnsNameList"=w328, "TableName"=w322) -> ("Update CMD"=w332:string)  [unwired: 7 in]
            "Update CMD 2" <- w332
            n96 = call-dynamic "SQL Execute.vi"("error in (no error)"=w330, "Return Data (T)"=FALSE, "Command Text"=w332, "HostDB in"=w331) -> ("error out"=w326:errorcluster, "HostDB out"=w327:refnum<class "SQLite.lvclass">)  [unwired: 3 in, 3 out]
            n97 = call-dynamic "Get Table Columns Name.vi"("error in (no error)"=w326, "TableName"=w322, "HostDB in"=w327) -> ("error out"=w321:errorcluster, "HostDB out"=w324:refnum<class "SQLite.lvclass">)  [unwired: 4 in, 3 out]
            n98 = call "Get ColumnName Alais Name.vi"("error in (no error)"=w321, "TableName"=w322, "SQLite in"=w324) -> ("error out"=w320:errorcluster, "SQLite out"=w323:refnum<class "SQLite.lvclass">)  [unwired: 6 in, 1 out]
          }
          frame True {
          }
        }
        n99 = call <vilib>:"Add State(s) to Queue__JKI_lib_State_Machine.vi"("State(s) in Front (\"\")"="UpdateNewResult" ("State(s) in Front (\"\")"), "State(s) in (\"\")"=w287) -> ("States Out"=w288:string)  [unwired: 13 in]
      }
      frame "UpdateNewResult" {
        # "更新新的列名称alais到ColumnName这一行。"
        n100 = property class="SQLite.lvclass"(reference=w381) -> (reference out=w374:refnum<class "SQLite.lvclass">, "Property:Alais_ColunmsList"=w372:string[], "Property:Table_ColunmsList"=w344:string[])  [unwired: 1 in, 1 out]
        n101 = call <userlib>:"StringToArray_Sushu.vi"("State Queue"=w371) -> ("Array"=w377:string[])  [unwired: 7 in, 3 out]
        n102 = call <userlib>:"StringToArray_Sushu.vi"("State Queue"=w361) -> ("Array"=w360:string[])  [unwired: 7 in, 3 out]
        n103 = Search 1D Array(1D array=w344, element="Result") -> (index of element=w375:i32)  [unwired: 1 in]
        n104 = Build Array (concatenate)(w359, w360) -> (w358:string[])
        n105 = for {
          tunnel: w377 -> [w386] mode=indexing
          tunnel: w372 -> [w388]
          tunnel: w375 -> [w387]
          tunnel: w344 -> [w385]
          tunnel: [w383] -> w356 mode=indexing
          n106 = Search 1D Array(1D array=w388, element=w386, start index (0)=w387) -> (index of element=w384:i32)
          n107 = Index Array(array=w385, index=w384) -> (element=w383:string)
        }
        n108 = Index Array(array=w344, index #1=1 ("index")) -> (element #1=w353:string, element #2=w352:string, element #3=w351:string)  [unwired: 2 in]
        n109 = Build Array("0" ("element"), w343, w342) -> (w348:string[])
        n110 = Build Array(w353, w352, w351) -> (w350:string[])
        n111 = call <userlib>:"Build string_ColumnsName=ColumnsValue_Where and.vi"("DB Type"=T2."SQLite", "ColumnsValue"=w348, "Check ASCII?"=FALSE, "ColumnsNameList"=w350) -> ("ColumnName='ColumnValue'"=w345:string)  [unwired: 7 in]
        n112 = Build Array (concatenate)("Result" ("TableName"), w356) -> (w357:string[])
        n113 = call <userlib>:"SQL_Update DB Table.vi"("where name='value'"=w345, "ColumnsValue"=w358, "ColumnsNameList"=w357, "TableName"=w368) -> ("Update CMD"=w364:string)  [unwired: 7 in]
        "Update CMD 3" <- w364
        n114 = call-dynamic "SQL Execute.vi"("error in (no error)"=w373, "Return Data (T)"=FALSE, "Command Text"=w364, "HostDB in"=w374) -> ("error out"=w362:errorcluster, "HostDB out"=w363:refnum<class "SQLite.lvclass">)  [unwired: 3 in, 3 out]
        n115 = call-dynamic "Get Table Columns Name.vi"("error in (no error)"=w362, "TableName"=w368, "HostDB in"=w363) -> ("error out"=w369:errorcluster, "HostDB out"=w370:refnum<class "SQLite.lvclass">)  [unwired: 4 in, 3 out]
        n116 = call <vilib>:"Add State(s) to Queue__jki_lib_state_machine.vi"("State(s) in (\"\")"=w366) -> ("States Out"=w367:string)  [unwired: 14 in]
      }
      frame "Update" {
        n117 = Unbundle By Name(w403) -> ("ResultStartindex"=w402:i32, "EmptyResultColumnIndex"=w401:i32)
        n118 = Index Array(array=w394, index #1=1 ("index")) -> (element #1=w417:string, element #2=w416:string, element #3=w415:string)  [unwired: 2 in]
        n119 = call <userlib>:"StringToArray_Sushu.vi"("State Queue"=w404) -> ("Array"=w398:string[], "Final size(s)"=w397:i32)  [unwired: 7 in, 2 out]
        n120 = Build Array("0" ("element"), w426, w425) -> (w412:string[])
        n121 = Build Array(w417, w416, w415) -> (w414:string[])
        n122 = Add(x=w402, y=w401) -> (x+y=w399:i32)
        n123 = Array Subset(array=w394, index=w399, length=w397) -> (w400:string[])
        n124 = call <userlib>:"Build string_ColumnsName=ColumnsValue_Where and.vi"("DB Type"=T2."SQLite", "ColumnsValue"=w412, "Check ASCII?"=FALSE, "ColumnsNameList"=w414) -> ("ColumnName='ColumnValue'"=w419:string)  [unwired: 7 in]
        n125 = Build Array (concatenate)(w391, w398) -> (w392:string[])
        n126 = Build Array (concatenate)("Result" ("Name"), w400) -> (w390:string[])
        n127 = call <userlib>:"SQL_Update DB Table.vi"("where name='value'"=w419, "ColumnsValue"=w392, "ColumnsNameList"=w390, "TableName"=w427) -> ("Update CMD"=w406:string)  [unwired: 7 in]
        "Update CMD" <- w406
        n128 = call-dynamic "SQL Execute.vi"("error in (no error)"=w396, "Return Data (T)"=FALSE, "Command Text"=w406, "HostDB in"=w424) -> ("error out"=w395:errorcluster, "HostDB out"=w423:refnum<class "SQLite.lvclass">)  [unwired: 3 in, 3 out]
        n129 = call <vilib>:"Add State(s) to Queue__jki_lib_state_machine.vi"("State(s) in (\"\")"=w420) -> ("States Out"=w421:string)  [unwired: 14 in]
        n130 = call <vilib>:"Add State(s) to Queue__jki_lib_state_machine.vi"("State(s) in Front (\"\")"=w405, "State(s) in (\"\")"=w406) -> ("States Out"=w407:string)  [unwired: 13 in]
        n131 = call <vilib>:"Add State(s) to Queue__jki_lib_state_machine.vi"("State(s) in (\"\")"=w408, "State(s) at Back (\"\")"=w407) -> ("States Out"=w409:string)  [unwired: 13 in]
      }
      frame "Close" {
        n132 = call-dynamic "Close Connection.vi"("error in (no error)"=w431, "HostDB in"=w429) -> ("error out"=w430:errorcluster, "HostDB out"=w428:refnum<class "SQLite.lvclass">)  [unwired: 8 in]
      }
    }
  }
  "error out" <- w3
  "CMD" <- w7
  n133 = Random Number (0-1)() -> (number: 0 to 1=→"number (0 to 1)":dbl)
